vi "DisplayTestItemData.vi"(8 "RowsData":string[](array[string])=["VoltageTest0", "电压测试0", "20", "12.000", "15", "VDC", "FAIL"], 9 "ID":dbl, 10 "real report 3":refnum<vi>, 11 "TEST 2":refnum<vi>) -> (2 "real report 3":refnum<vi>, 3 "TEST 2":refnum<vi>)   [LabVIEW 2018]
uses:
  <vilib>/Utility/miscctls.llb/LVRowAndColumnTypeDef.ctl
panel:
  out "添加的数组 2":string[][](array[string])
  out "添加的数组":string[][](array[string])
  in  "TEST":i32(listbox)
  in  "real report 2":i32(listbox) caption="real report"
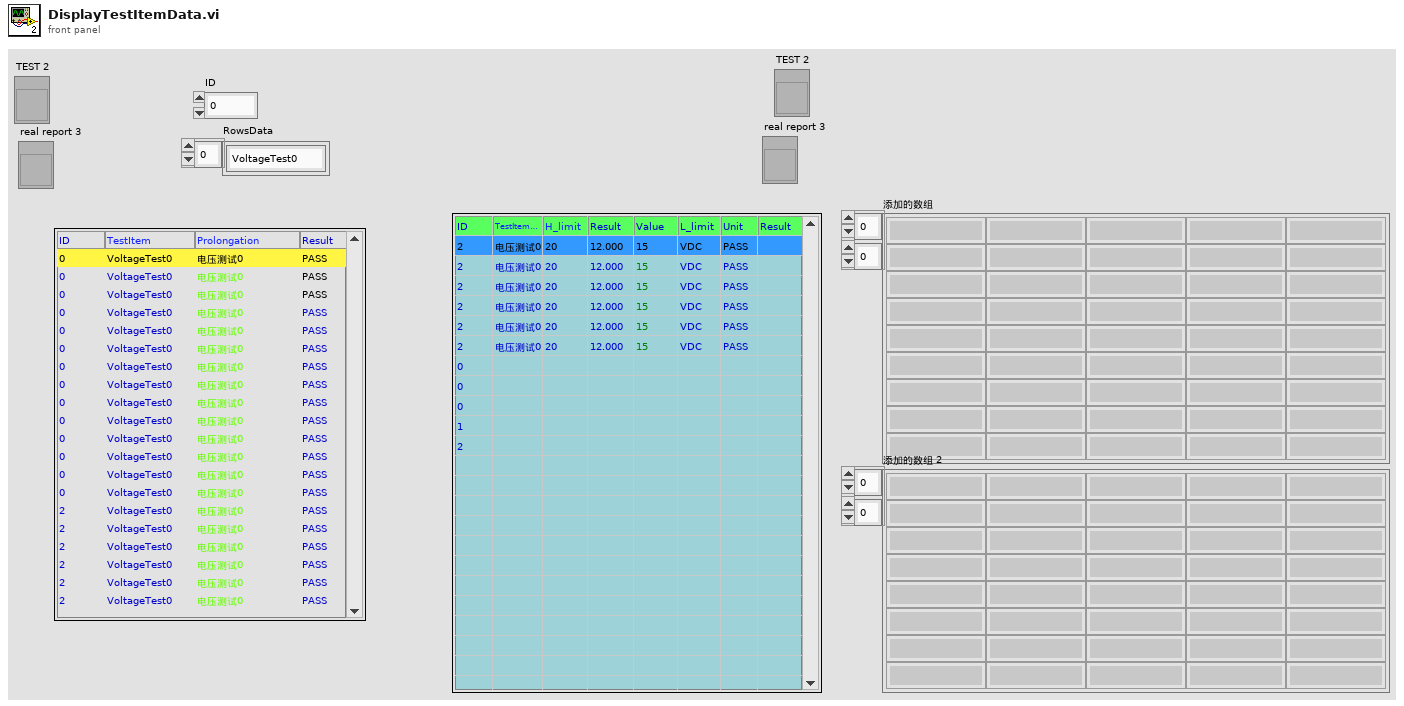
[diagram p1: front panel]
types:
  T1 = typedef "LVRowAndColumnTypeDef.ctl" = cluster{"Row":i32, "Column":i32}
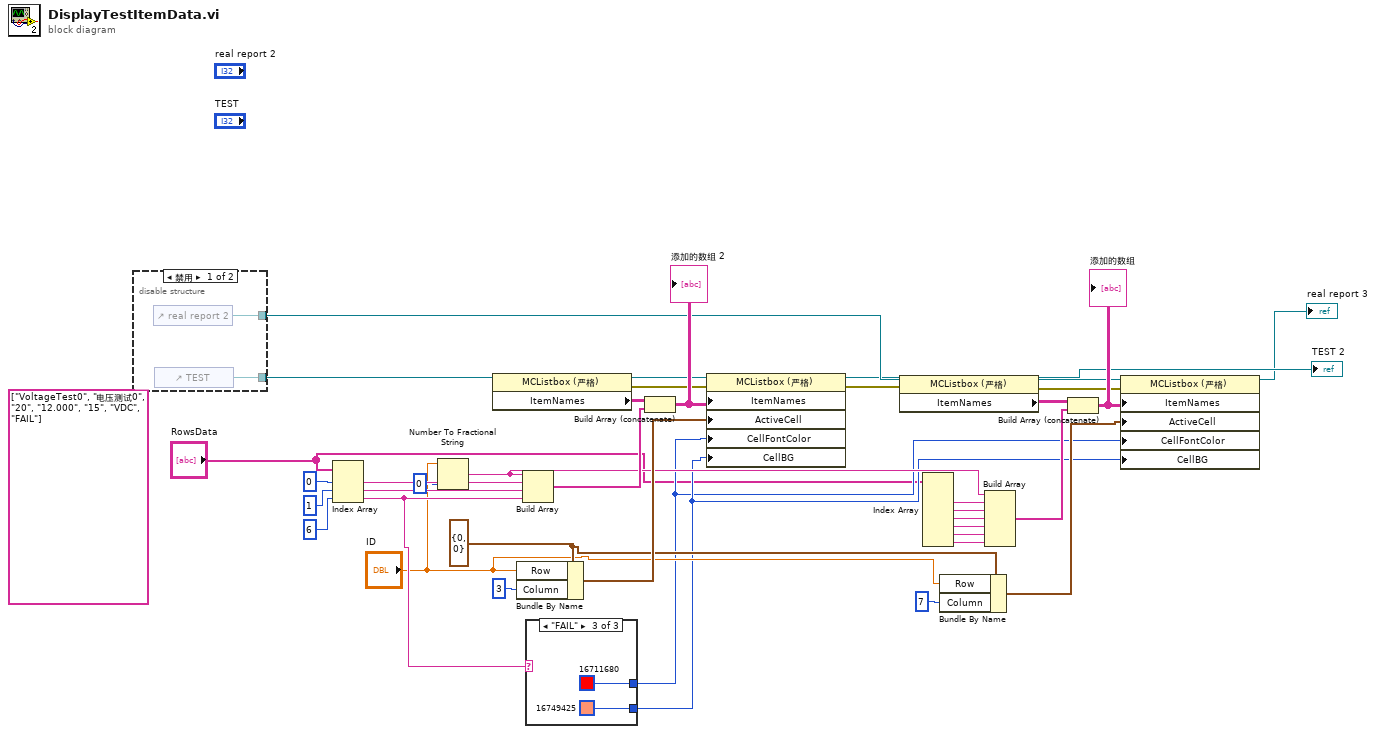
[diagram p0: block diagram]
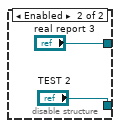
[diagram p2: hidden frame]
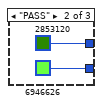
[diagram p4: hidden frame]
diagram:
  w8 = T1 {"Row"=0, "Column"=0} ("活动单元格:活动单元格")
  (unwired) string[] ["VoltageTest0", "电压测试0", "20", "12.000", "15", "VDC", "FAIL"]
  n1 = disable-structure shown="禁用" {
    disable-tunnel: [w40 "TEST 2"] -> w30
    disable-tunnel: [w39 "real report 3"] -> w24
    frame Disabled {
      n2 = control-ref of="real report 2"() -> (w39:refnum<vi>)
      n3 = control-ref of="TEST"() -> (w40:refnum<vi>)
    }
    frame Enabled {
    }
  }
  n4 = Index Array(array="RowsData", index #1=0 ("索引"), index #2=1 ("索引"), index #3=6 ("索引")) -> (element #1=w35:string, element #2=w34:string, element #3=w25:string)
  n5 = Number To Fractional String(number="ID", precision (6)=i16 0 ("精度(6)")) -> (F-format string=w20:string)  [unwired: 2 in]
  n6 = property class="MCListbox (严格)"(reference=w30) -> (reference out=w26:refnum<vi>, error out=w10:errorcluster, "ItemNames"=w33:string[][])  [unwired: 1 in]
  n7 = Bundle By Name(cluster=w8, "Row"="ID", "Column"=3) -> (w28:T1)
  n8 = Build Array(w20, w35, w34, w25) -> (w32:string[])
  n9 = case shown="\"FAIL\"" w25 {
    tunnel: [_ u32 2853120 u32 16711680] -> w4
    tunnel: [_ u32 6946626 u32 16749425] -> w5
    frame "假", Default {
    }
    frame "PASS" {
    }
    frame "FAIL" {
    }
  }
  n10 = Build Array (concatenate)(w33, w32) -> (w31:string[][])
  "添加的数组 2" <- w31
  n11 = property class="MCListbox (严格)"(reference=w26, error in=w10, "ItemNames"=w31, "ActiveCell"=w28, "CellFontColor"=w4, "CellBG"=w5) -> (reference out=→"TEST 2":refnum<vi>, error out=w23:errorcluster)
  n12 = property class="MCListbox (严格)"(reference=w24, error in=w23) -> (reference out=w12:refnum<vi>, error out=w11:errorcluster, "ItemNames"=w21:string[][])
  n13 = Index Array(array="RowsData") -> (element #2=w19:string, element #3=w18:string, element #4=w17:string, element #5=w16:string, element #6=w15:string, element #7=w14:string)  [unwired: 7 in, 1 out]
  n14 = Bundle By Name(cluster=w8, "Row"="ID", "Column"=7) -> (w6:T1)
  n15 = Build Array(w20, w19, w18, w17, w16, w15, w14) -> (w13:string[])
  n16 = Build Array (concatenate)(w21, w13) -> (w22:string[][])
  "添加的数组" <- w22
  n17 = property class="MCListbox (严格)"(reference=w12, error in=w11, "ItemNames"=w22, "ActiveCell"=w6, "CellFontColor"=w4, "CellBG"=w5) -> (reference out=→"real report 3":refnum<vi>)  [unwired: 1 out]
